vi "Mining and Dumping.vi"() -> ()   [LabVIEW 2015]
uses:
  <vilib>/myRIO/Instrument Drivers/Onboard IO/PWM/typedefs/PWM Reference.ctl
  <vilib>/myRIO/Common/Instrument Driver Framework/Utilities/typedefs/myRIO Generic Hardware Reference.ctl
  <vilib>/myRIO/Common/Instrument Driver Framework/Utilities/typedefs/Hardware Version Enum.ctl
  <vilib>/myRIO/Common/Instrument Driver Framework/Utilities/typedefs/myRIO v1.0 Reference.ctl
  <vilib>/myRIO/Common/Instrument Driver Framework/Utilities/typedefs/Generic FPGA Reference.ctl
  <vilib>/myRIO/Common/Instrument Driver Framework/myRIO v1.0/PWM/typedefs/PWM Channels Enum.ctl
  <vilib>/myRIO/Instrument Drivers/Onboard IO/PWM/typedefs/PWM Configuration.ctl
  <vilib>/userdefined/High Color/nirio_resource_hc.ctl
  <vilib>/myRIO/Instrument Drivers/Onboard IO/AI/typedefs/AI Reference.ctl
  <vilib>/myRIO/Common/Instrument Driver Framework/myRIO v1.0/AI/typedefs/AI Channels List.ctl
  <vilib>/myRIO/Common/Instrument Driver Framework/myRIO v1.0/AI/typedefs/AI Channels Enum.ctl
  <vilib>/myRIO/Common/Instrument Driver Framework/Utilities/typedefs/Analog Scaling Constants List.ctl
  <vilib>/myRIO/Common/Instrument Driver Framework/Utilities/typedefs/Analog Scaling Constants.ctl
  <vilib>/myRIO/Common/Instrument Driver Framework/Utilities/vis/Is FPGA Ref Available.vi
  <vilib>/myRIO/Common/Instrument Driver Framework/myRIO v1.0/PWM/vis/myRIO v1.1 Open PWM.vi
  <vilib>/myRIO/Instrument Drivers/Onboard IO/PWM/vis/Set Duty Cycle and Frequency.vi
  <vilib>/myRIO/Common/Instrument Driver Framework/myRIO v1.0/AI/vis/myRIO v1.1 Open AI.vi
  <vilib>/myRIO/Instrument Drivers/Onboard IO/AI/vis/Read.vi
  <vilib>/myRIO/Common/Instrument Driver Framework/Utilities/vis/Validate Channels.vi
  <vilib>/myRIO/Common/Instrument Driver Framework/myRIO v1.0/PWM/vis/myRIO v1.0 Reserve PWM.vi
  <vilib>/myRIO/Common/Instrument Driver Framework/myRIO v1.0/AI/vis/myRIO v1.0 Reserve AI.vi
  <vilib>/myRIO/Common/Instrument Driver Framework/myRIO v1.0/PWM/vis/myRIO v1.0 Build MUX Configuration PWM.vi
  <vilib>/myRIO/Common/Instrument Driver Framework/myRIO v1.0/Resource Manager/vis/myRIO v1.0 Reserve Channel List.vi
  <vilib>/myRIO/Common/Instrument Driver Framework/myRIO v1.0/AI/vis/myRIO v1.0 Build MUX Configuration AI.vi
  <vilib>/myRIO/Common/Instrument Driver Framework/myRIO v1.0/Resource Manager/vis/myRIO v1.0 Create Configuration List.vi
  <vilib>/myRIO/Common/Instrument Driver Framework/myRIO v1.0/Resource Manager/vis/myRIO v1.0 Reserve Channel.vi
  <vilib>/myRIO/Common/Instrument Driver Framework/myRIO v1.0/Resource Manager/vis/myRIO v1.0 Unreserve Channel.vi
  <vilib>/myRIO/Common/Instrument Driver Framework/myRIO v1.0/Resource Manager/vis/myRIO v1.0 Build Mutex Name.vi
  <vilib>/Utility/VariantDataType/GetNumericInfo.vi
  <vilib>/Utility/error.llb/Error Cluster From Error Code.vi
  <vilib>/myRIO/Common/Instrument Driver Framework/myRIO v1.0/myRIO v1.1 Open.vi
  <vilib>/myRIO/Common/Instrument Driver Framework/Utilities/vis/IO Manager.vi
  <vilib>/myRIO/Common/Instrument Driver Framework/Utilities/vis/Configuration Manager.vi
  <vilib>/myRIO/Common/Instrument Driver Framework/myRIO v1.0/Resource Manager/vis/myRIO v1.0 Configure IO.vi
  <vilib>/myRIO/Common/Instrument Driver Framework/myRIO v1.0/myRIO v1.0 Close.vi
  <vilib>/myRIO/Common/Instrument Driver Framework/myRIO v1.0/PWM/vis/myRIO v1.0 Write PWM.vi
  <vilib>/myRIO/Common/Instrument Driver Framework/myRIO v1.0/AI/vis/myRIO v1.0 Get Scaling Constants AI.vi
  <vilib>/myRIO/Common/Instrument Driver Framework/myRIO v1.0/AI/vis/myRIO v1.0 Read AI.vi
  <vilib>/myRIO/Express VI/Onboard IO/PWM/PWM Express VI.xnode
  <vilib>/myRIO/Instrument Drivers/Onboard IO/PWM/vis/myRIO PWM Open.xnode
  <vilib>/myRIO/Express VI/Onboard IO/AI/AI Express VI.xnode
  <vilib>/myRIO/Instrument Drivers/Onboard IO/AI/vis/myRIO AI Open.xnode
  <vilib>/myRIO/Instrument Drivers/Onboard IO/PWM/PWM.lvlib
  <vilib>/myRIO/Instrument Drivers/Onboard IO/AI/AI.lvlib
panel:
  in  "stop":bool
  out "Servo Stop":i64
  out "Stop":bool
  in  "Numeric":i32
  out "Full":bool
  out "A/AI0 (Pin 3) 2":dbl
  out "A/AI0 (Pin 3)":dbl
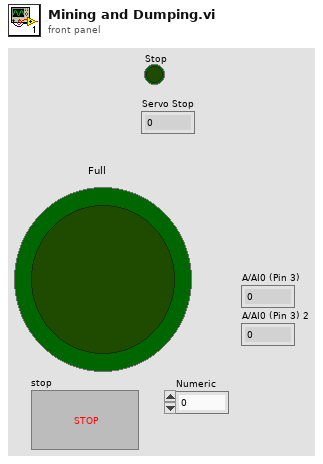
[diagram p1: front panel]
types:
  T1 = typedef "PWM.lvlib/PWM Reference.ctl" = cluster{"myRIO Reference":T2, "PWM Channels Enum":T6, "PWM Configuration":T7}
  T2 = typedef "myRIO Generic Hardware Reference.ctl" = cluster{"myRIO Model":T3, "myRIO Hardware Reference":T4}
  T3 = typedef "Hardware Version Enum.ctl" = enum16{"Unknown", "myRIO-1900", "myRIO-1950", "roboRIO"}
  T4 = typedef "myRIO v1.0 Reference.ctl" = cluster{"Generic FPGA Reference":T5, "Allow multiple opens":bool}
  T5 = typedef "Generic FPGA Reference.ctl" = refnum<k20>
  T6 = typedef "PWM Channels Enum.ctl" = enum16{"Not Connected", "C/PWM0", "C/PWM1", "A/PWM0", "A/PWM1", "A/PWM2", "B/PWM0", "B/PWM1", "B/PWM2", "PWM/PWM0", "PWM/PWM1", "PWM/PWM2", "PWM/PWM3", "PWM/PWM4", "PWM/PWM5", "PWM/PWM6", "PWM/PWM7", "PWM/PWM8", "PWM/PWM9"}
  T7 = typedef "PWM.lvlib/PWM Configuration.ctl" = cluster{"Frequency":dbl, "Duty Cycle":dbl}
  T8 = typedef "nirio_resource_hc.ctl" = tag
  T9 = typedef "AI.lvlib/AI Reference.ctl" = cluster{"myRIO Reference":T2, "AI Channels List":T10, "AI Scaling Constants List":T12}
  T10 = typedef "AI Channels List.ctl" = T11[]
  T11 = typedef "AI Channels Enum.ctl" = enum16{"Not Connected", "AudioIn/Left", "AudioIn/Right", "C/AI0", "C/AI1", "A/AI0", "A/AI1", "A/AI2", "A/AI3", "B/AI0", "B/AI1", "B/AI2", "B/AI3", "AI/AI0", "AI/AI1", "AI/AI2", "AI/AI3"}
  T12 = typedef "Analog Scaling Constants List.ctl" = T13[]
  T13 = typedef "Analog Scaling Constants.ctl" = cluster{"LSB Weight (Volts)":dbl, "Offset (Volts)":dbl, "Signed?":bool}
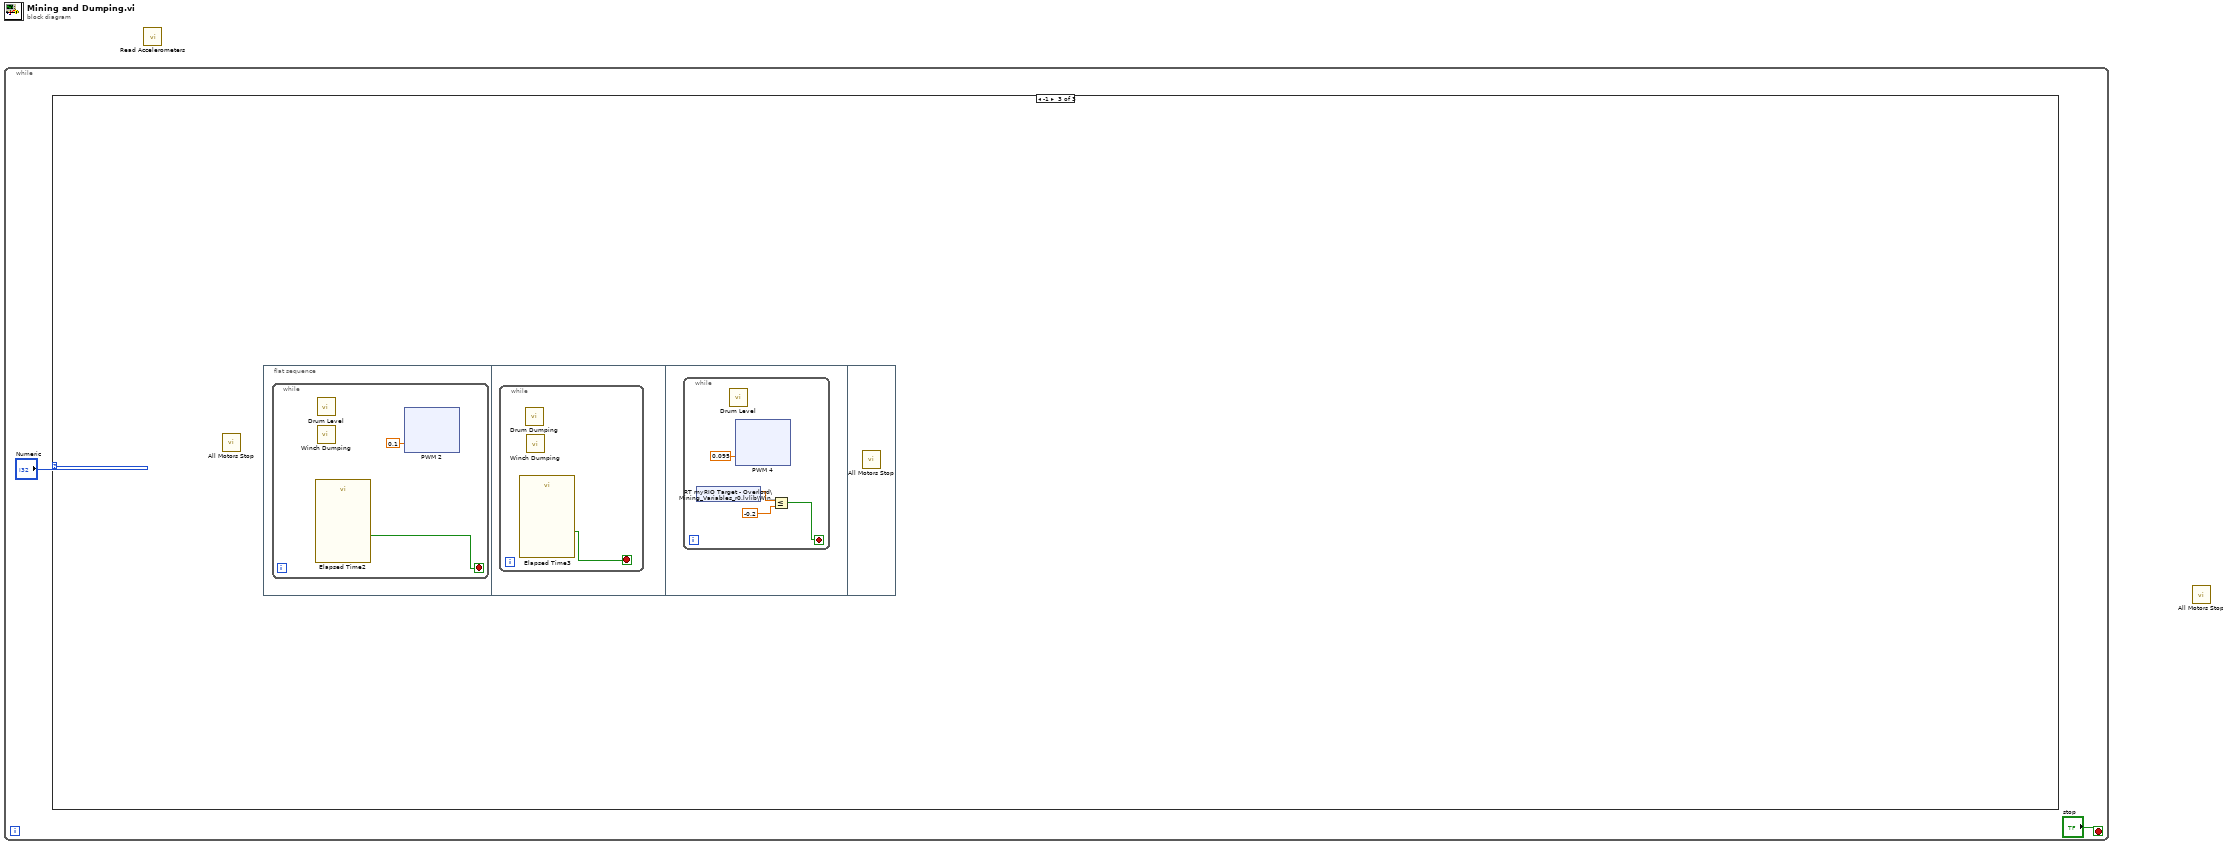
[diagram p0: block diagram]
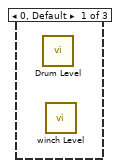
[diagram p2: hidden frame]
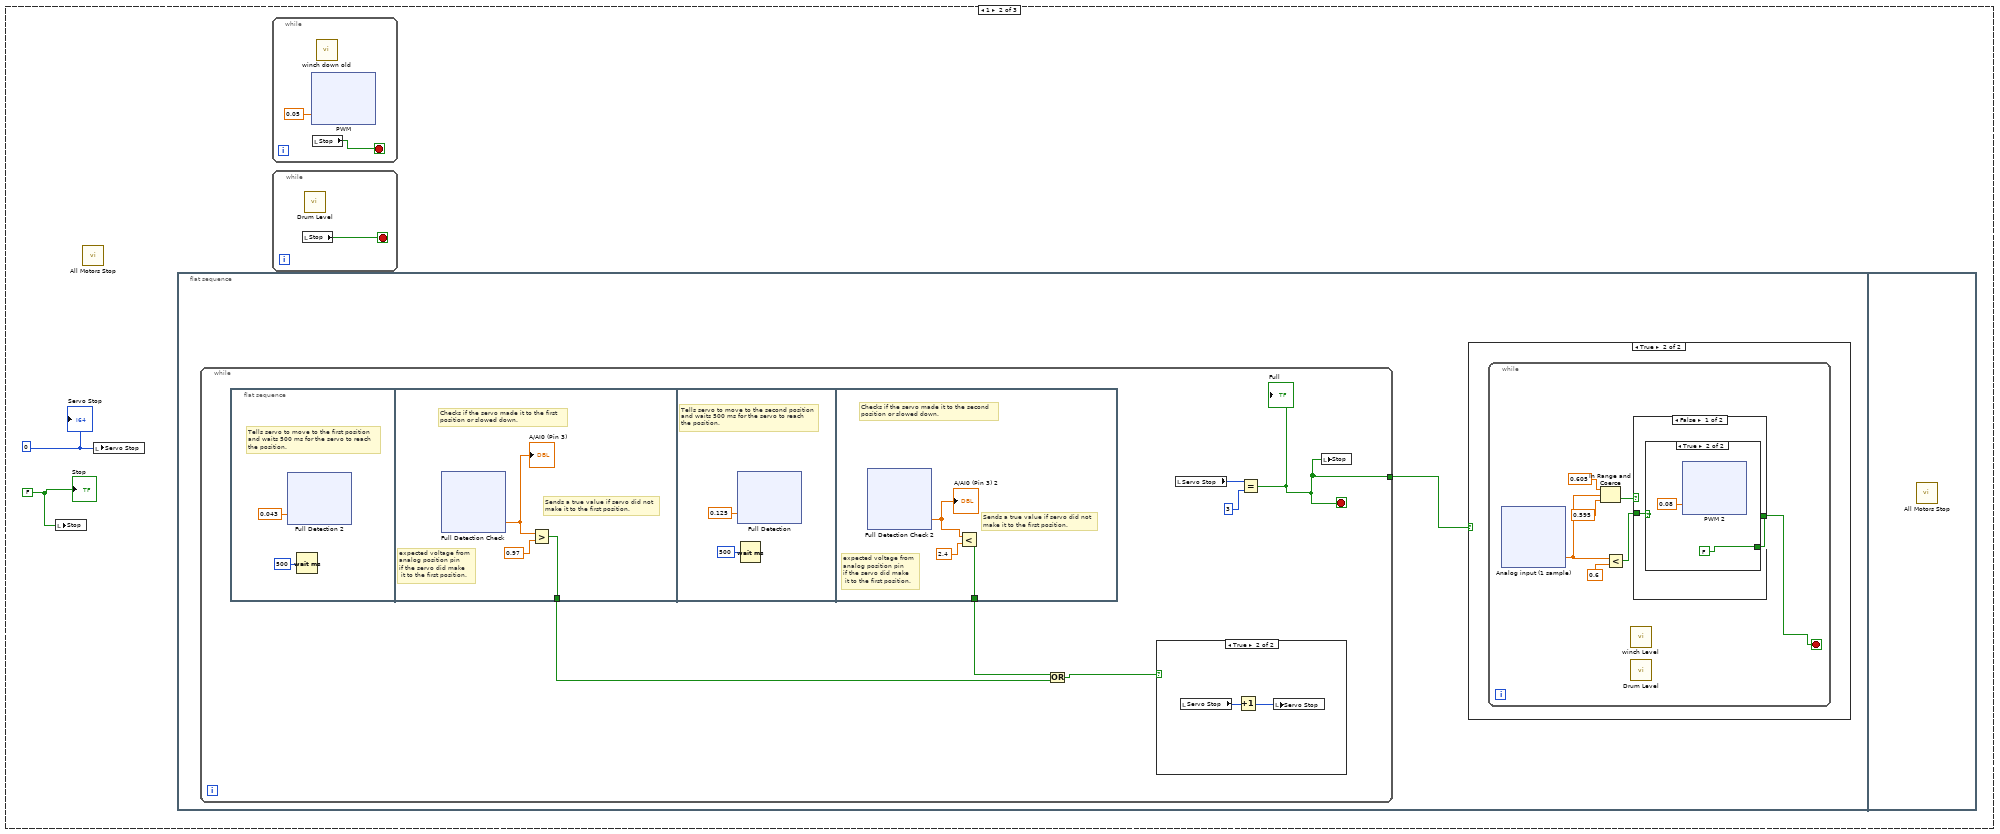
[diagram p3: hidden frame]
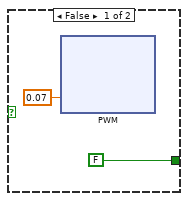
[diagram p5: hidden frame]
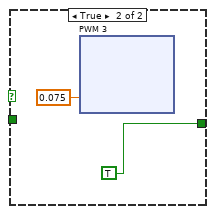
[diagram p6: hidden frame]
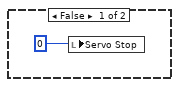
[diagram p7: hidden frame]
diagram:
  n1 = while {
    stop <- "stop" stop-if-true
    n2 = case shown="-1" "Numeric" {
      frame 0, Default {
        n3 = call "Drum Level.vi"() -> ()  [unwired: 12 in]
        n4 = call "winch Level.vi"() -> ()  [unwired: 12 in]
      }
      frame 1 {
        w4 = FALSE ("Stop")
        w3 = i64 0 ("Servo Stop")
        n5 = local write "Stop"(w4) -> ()
        n6 = call "All Motors Stop.vi"() -> ()  [unwired: 12 in]
        n7 = local write "Servo Stop"(w3) -> ()
        n8 = flat-sequence {
          frame #0 {
            n9 = while {
              tunnel: [w200] -> w42
              stop <- w200 stop-if-true
              n10 = flat-sequence {
                tunnel: [w247] -> w203
                tunnel: [w323] -> w204
                frame #0 {
                  # "Tells servo to move to the first position\nand waits 500 ms for the servo to reach \nthe position."
                  n11 = xnode "Full Detection 2"("Duty Cycle"=0.043) -> ()  [unwired: 1 in, 1 out]
                  n12 = Wait (ms)(milliseconds to wait=u32 500) -> ()  [unwired: 1 out]
                }
                frame #1 {
                  # "Sends a true value if servo did not \nmake it to the first position."
                  # "expected voltage from \nanalog position pin \nif the servo did make\n it to the first position."
                  # "Checks if the servo made it to the first \nposition or slowed down."
                  n13 = xnode "Full Detection Check"() -> ("A/AI0 (Pin 3)"=w246:dbl)  [unwired: 1 in, 1 out]
                  "A/AI0 (Pin 3)" <- w246
                  n14 = Greater?(x=w246, y=0.97) -> (0:w247:bool)
                }
                frame #2 {
                  # "Tells servo to move to the second position\nand waits 500 ms for the servo to reach \nthe position."
                  n15 = xnode "Full Detection"("Duty Cycle"=0.125) -> ()  [unwired: 1 in, 1 out]
                  n16 = Wait (ms)(milliseconds to wait=u32 500) -> ()  [unwired: 1 out]
                }
                frame #3 {
                  # "Sends a true value if servo did not \nmake it to the first position."
                  # "expected voltage from \nanalog position pin \nif the servo did make\n it to the first position."
                  # "Checks if the servo made it to the second \nposition or slowed down."
                  n17 = xnode "Full Detection Check 2"() -> ("A/AI0 (Pin 3)"=w325:dbl)  [unwired: 1 in, 1 out]
                  "A/AI0 (Pin 3) 2" <- w325
                  n18 = Less?(x=w325, y=2.4) -> (x < y?=w323:bool)
                }
              }
              n19 = Or(x=w204, y=w203) -> (x .or. y?=w205:bool)
              n20 = case shown="True" w205 {
                frame False {
                  n21 = local write "Servo Stop"(i64 0 ("Servo Stop")) -> ()
                }
                frame True {
                  n22 = local read "Servo Stop"() -> (w208:i64)
                  n23 = Increment(x=w208) -> (x+1=w207:i64)
                  n24 = local write "Servo Stop"(w207) -> ()
                }
              }
              n25 = local read "Servo Stop"() -> (w201:i64)
              n26 = Equal?(x=w201, y=i64 3) -> (x = y?=w200:bool)
              "Full" <- w200
              n27 = local write "Stop"(w200) -> ()
            }
            n28 = case shown="True" w42 {
              frame False {
              }
              frame True {
                n29 = while {
                  stop <- w43 stop-if-true
                  n30 = xnode "Analog input (1 sample)"() -> ("A/AI1 (Pin 5)"=w46:dbl)  [unwired: 1 in, 1 out]
                  n31 = In Range and Coerce(upper limit=0.605, x=w46, lower limit=0.595) -> (In Range?=w47:bool)  [unwired: 1 out]
                  n32 = Less?(x=w46, y=0.6) -> (x < y?=w48:bool)
                  n33 = call "winch Level.vi"() -> ()  [unwired: 12 in]
                  n34 = call "Drum Level.vi"() -> ()  [unwired: 12 in]
                  n35 = case shown="False" w47 {
                    tunnel: w48 -> [w51 _]
                    tunnel: [w50 TRUE] -> w43
                    frame False {
                      n36 = case shown="True" w51 {
                        tunnel: [FALSE FALSE] -> w50
                        frame False {
                          n37 = xnode "PWM"("Duty Cycle"=0.07) -> ()  [unwired: 1 in, 1 out]
                        }
                        frame True {
                          n38 = xnode "PWM 2"("Duty Cycle"=0.08) -> ()  [unwired: 1 in, 1 out]
                        }
                      }
                    }
                    frame True {
                      n39 = xnode "PWM 3"("Duty Cycle"=0.075) -> ()  [unwired: 1 in, 1 out]
                    }
                  }
                }
              }
            }
          }
          frame #1 {
            n40 = call "All Motors Stop.vi"() -> ()  [unwired: 12 in]
          }
        }
        n41 = while {
          stop <- w5 stop-if-true
          n42 = xnode "PWM"("Duty Cycle"=0.05) -> ()  [unwired: 1 in, 1 out]
          n43 = local read "Stop"() -> (w5:bool)
          n44 = call "winch down old.vi"() -> ()  [unwired: 12 in]
        }
        n45 = while {
          stop <- w363 stop-if-true
          n46 = local read "Stop"() -> (w363:bool)
          n47 = call "Drum Level.vi"() -> ()  [unwired: 12 in]
        }
        "Stop" <- w4
        "Servo Stop" <- w3
      }
      frame -1 {
        n48 = call "All Motors Stop.vi"() -> ()  [unwired: 12 in]
        n49 = flat-sequence {
          frame #0 {
            n50 = while {
              stop <- w365 stop-if-true
              n51 = call "Elapsed Time2"() -> ("Time has Elapsed"=w365:bool)  [unwired: 12 in, 7 out]
              n52 = call "Drum Level.vi"() -> ()  [unwired: 12 in]
              n53 = call "Winch Dumping.vi"() -> ()  [unwired: 12 in]
              n54 = xnode "PWM 2"("Duty Cycle"=0.1) -> ()  [unwired: 1 in, 1 out]
            }
          }
          frame #1 {
            n55 = while {
              stop <- w401 stop-if-true
              n56 = call "Elapsed Time3"() -> ("Time has Elapsed"=w401:bool)  [unwired: 12 in, 7 out]
              n57 = call "Drum Dumping.vi"() -> ()  [unwired: 12 in]
              n58 = call "Winch Dumping.vi"() -> ()  [unwired: 12 in]
            }
          }
          frame #2 {
            n59 = while {
              stop <- w404 stop-if-true
              n60 = shared-variable "RT myRIO Target - Overlord\\Mining_Variables_r0.lvlib\\Winch Accel x"() -> (w405:dbl)  [unwired: 1 in, 1 out]
              n61 = call "Drum Level.vi"() -> ()  [unwired: 12 in]
              n62 = xnode "PWM 4"("Duty Cycle"=0.095) -> ()  [unwired: 1 in, 1 out]
              n63 = Less Or Equal?(x=w405, y=-0.2) -> (x <= y?=w404:bool)
            }
          }
          frame #3 {
            n64 = call "All Motors Stop.vi"() -> ()  [unwired: 12 in]
          }
        }
      }
    }
  }
  n65 = call "Read Accelerometers.vi"() -> ()  [unwired: 11 in, 9 out]
  n66 = call "All Motors Stop.vi"() -> ()  [unwired: 12 in]
